vi "Get Class.vi"   [LabVIEW 2021, in "Omni_Bus.lvclass"]
uses:
  Omni_Bus.lvclass
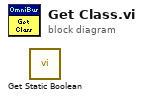
[diagram p0: block diagram]
diagram:
  n1 = call "Get Static Boolean.vi"() -> ()  [unwired: 9 in, 3 out]
